vi "CRYCall Protect Dll.vi"(0 "lp1":u32 format="%x", 1 "lp2":u32, 2 "p1":u16=33014 format="%x", 3 "p2":u16=7168 format="%x", 4 "p3":u16=18159 format="%x", 5 "p4":u16=18390 format="%x", 6 "handle":u16[](array[numeric]), 7 "buffer":u8[](array[numeric]), 8 "function":u16=1) -> (12 "return type":u16, 13 "buffer Out":u8[](array[numeric]), 14 "lp1 Out":u32 format="%x", 15 "lp2 Out":u32, 16 "p1 Out":u16=50252 format="%x", 17 "p2 Out":u16=51448 format="%x", 18 "p3 Out":u16=1945 format="%x", 19 "p4 Out":u16=50235 format="%x")   [LabVIEW 2013]
uses:
  Ry4S.dll
panel:
  # "12345678"
  # "sead"
  # "80F6"
  # "1C00"
  # "46EF"
  # "47D6"
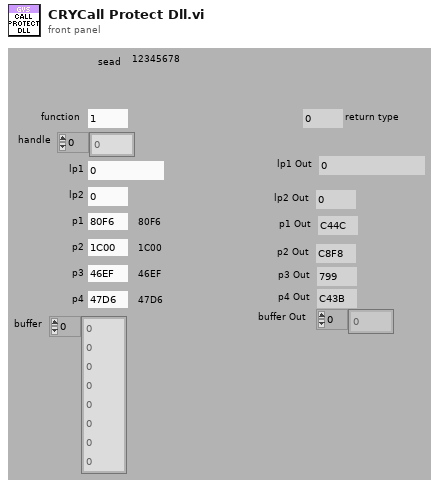
[diagram p1: front panel]
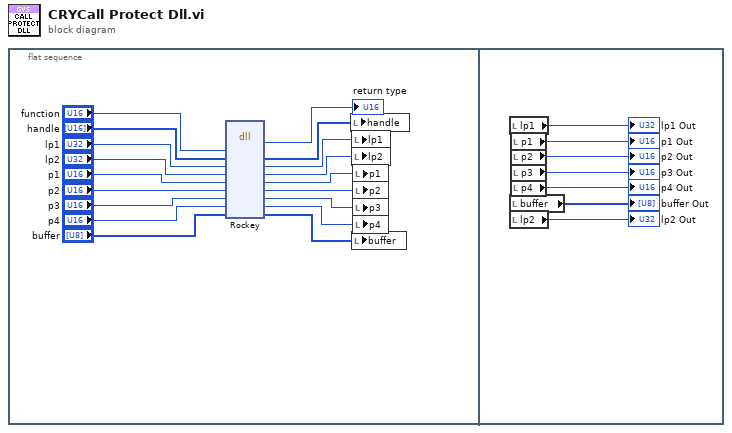
[diagram p0: block diagram]
diagram:
  n1 = flat-sequence {
    frame #0 {
      n2 = dll-call lib="D:/LabView_Project/CRY6181/Ry4S.dll" fn="Rockey"("function"="function", "handle"="handle", "lp1"="lp1", "lp2"="lp2", "p1"="p1", "p2"="p2", "p3"="p3", "p4"="p4", "buffer"="buffer") -> ("return type"=→"return type":u16, "handle"=w1:u16[], "lp1"=w10:u32, "lp2"=w9:u32, "p1"=w8:u16, "p2"=w7:u16, "p3"=w6:u16, "p4"=w5:u16, "buffer"=w2:u8[])  [unwired: 4 in, 2 out]
      n3 = local write "handle"(w1) -> ()
      n4 = local write "lp1"(w10) -> ()
      n5 = local write "lp2"(w9) -> ()
      n6 = local write "buffer"(w2) -> ()
      n7 = local write "p1"(w8) -> ()
      n8 = local write "p2"(w7) -> ()
      n9 = local write "p3"(w6) -> ()
      n10 = local write "p4"(w5) -> ()
    }
    frame #1 {
      n11 = local read "lp1"() -> (→"lp1 Out":u32)
      n12 = local read "buffer"() -> (→"buffer Out":u8[])
      n13 = local read "lp2"() -> (→"lp2 Out":u32)
      n14 = local read "p1"() -> (→"p1 Out":u16)
      n15 = local read "p2"() -> (→"p2 Out":u16)
      n16 = local read "p3"() -> (→"p3 Out":u16)
      n17 = local read "p4"() -> (→"p4 Out":u16)
    }
  }
